vi "Do.vi"(6 "Input":variant, 8 "error in":errorcluster, 9 "Self Enqueuer":refnum<class "Message Enqueuer.lvclass">, 10 "Series Enqueuer":refnum<class "Message Enqueuer.lvclass">, 11 "Sample Watertemp PWM Control in":refnum<class "Sample Watertemp PWM Control.lvclass">) -> (0 "error out":errorcluster, 3 "Sample Watertemp PWM Control out":refnum<class "Sample Watertemp PWM Control.lvclass">)   [LabVIEW 2023, in "Sample Watertemp PWM Control.lvclass"]
uses:
  Sample Watertemp PWM Control.lvclass
  <vilib>/ActorFramework/Message Enqueuer/Message Enqueuer.lvclass
  Task/Task Base/Task Base.lvclass/Task Base.ctl
  Sample Watertemp PWM Control.lvclass/Sample Watertemp PWM Control.ctl
  Task/Task Base/Task Base.lvclass
  Measure and Stimulus Subsystems/Measure and Stimulus Subsystems.lvclass
  D:/git/HAL/HAL GOOP4/Task/Task Base/Task Base.lvclass
  D:/git/HAL/HAL GOOP4/Tests/RT Tests/Sample Tasks/Sample Watertemp PWM Control/Sample Watertemp PWM Control.lvclass
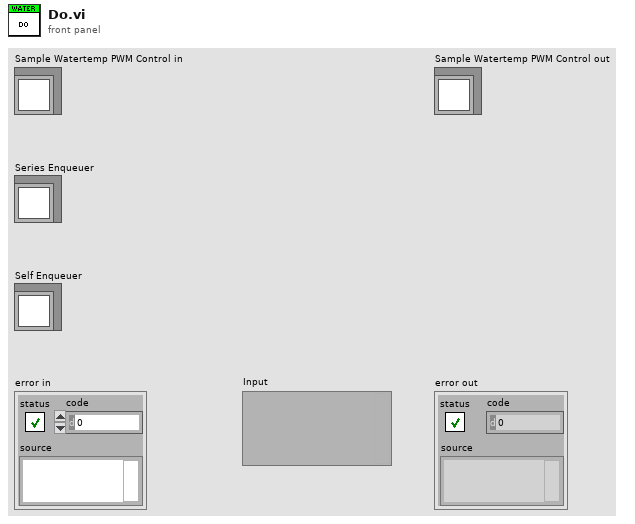
[diagram p1: front panel]
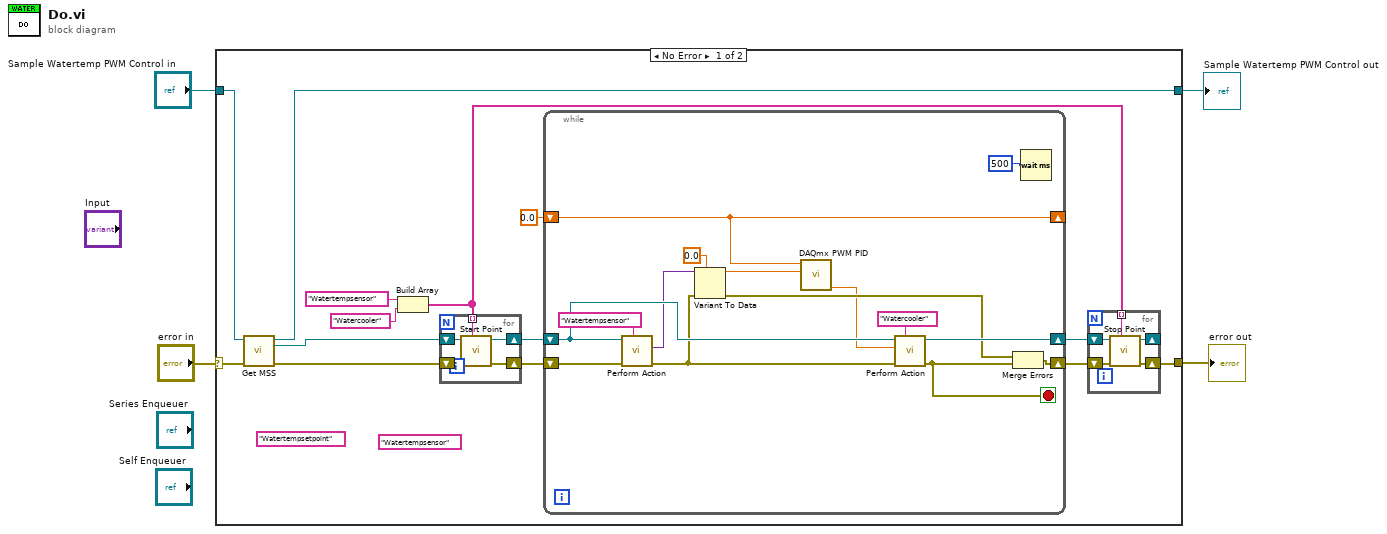
[diagram p0: block diagram]
diagram:
  n1 = case shown="No Error" "error in" {
    selector: "error in" -> [w15 w45]
    tunnel: [w11 w45] -> w1
    tunnel: [w7 w44] -> w4
    tunnel: "Sample Watertemp PWM Control in" -> [w6 w44]
    frame No Error {
      (unwired) "Watertempsetpoint" ("Target Name")
      (unwired) "Watertempsensor" ("Target Identifier")
      n2 = call "Get MSS.vi"("error in (no error)"=w15, "Task Base in"=w6) -> ("error out"=w14:errorcluster, "MSS"=w13:refnum<class "Measure and Stimulus Subsystems.lvclass">, "Task Base out"=w7:refnum<class "Sample Watertemp PWM Control.lvclass">)  [unwired: 7 in]
      n3 = Build Array("Watertempsensor" ("Target Identifier"), "Watercooler" ("Target Identifier")) -> (w8:string[])
      n4 = for {
        shift-right: [w23] -> w18
        shift-left: w14 -> [w21]
        shift-right: [w22] -> w17
        shift-left: w13 -> [w20]
        tunnel: w8 -> [w19] mode=indexing
        n5 = call "Start Point.vi"("Point Ident"=w19, "error in"=w21, "MSS in"=w20) -> ("error out"=w23:errorcluster, "MSS out"=w22:refnum<class "Measure and Stimulus Subsystems.lvclass">)  [unwired: 7 in]
      }
      n6 = while {
        shift-right: [w32] -> w16
        shift-left: w18 -> [w34]
        shift-right: [w36] -> w12
        shift-left: w17 -> [w33]
        shift-right: [w28] -> _
        shift-left: 0.0 -> [w28]
        stop <- w27 stop-if-true
        n7 = call "Perform Action.vi"("Point Ident"="Watertempsensor" ("Target Identifier"), "error in"=w34, "MSS in"=w33) -> ("error out"=w29:errorcluster, "Output"=w30:variant)  [unwired: 6 in, 1 out]
        n8 = Variant To Data(error in=w29, type=0.0, Variant=w30) -> (data=w25:dbl, error out=w26:errorcluster)
        n9 = call "DAQmx PWM PID.vi"("Process Variable"=w25, "Setpoint"=w28) -> ("Control Output"=w24:dbl)  [unwired: 9 in]
        n10 = call "Perform Action.vi"("Point Ident"="Watercooler" ("Target Ident"), "error in"=w29, "Input"=w24, "MSS in"=w33) -> ("error out"=w27:errorcluster, "MSS out"=w36:refnum<class "Measure and Stimulus Subsystems.lvclass">)  [unwired: 5 in, 1 out]
        n11 = Merge Errors(w26, w27) -> (w32:errorcluster)
        n12 = Wait (ms)(milliseconds to wait=u32 500) -> ()  [unwired: 1 out]
      }
      n13 = for {
        shift-right: [w41] -> w11
        shift-left: w16 -> [w43]
        tunnel: w8 -> [w39] mode=indexing
        shift-right: [w40] -> _
        shift-left: w12 -> [w42]
        n14 = call "Stop Point.vi"("Point Ident"=w39, "error in"=w43, "MSS in"=w42) -> ("error out"=w41:errorcluster, "MSS out"=w40:refnum<class "Measure and Stimulus Subsystems.lvclass">)  [unwired: 7 in]
      }
    }
    frame Error {
    }
  }
  "error out" <- w1
  "Sample Watertemp PWM Control out" <- w4
